vi "SubPanelRef.vi"(0 "reference":refnum<vi>, 11 "error in":errorcluster) -> (4 "reference out":refnum<vi>, 8 "InsertedVI":refnum<vi>, 15 "error out":errorcluster)   [LabVIEW 2016]
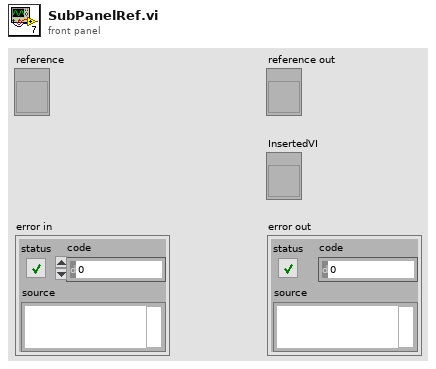
[diagram p1: front panel]
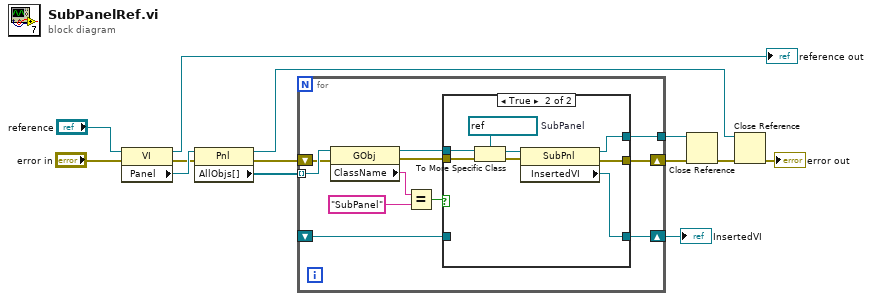
[diagram p0: block diagram]
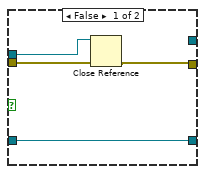
[diagram p2: hidden frame]
diagram:
  n1 = property class="VI"(reference="reference", error in="error in") -> (reference out=→"reference out":refnum<vi>, error out=w9:errorcluster, "Panel"=w13:refnum<vi>)
  n2 = property class="Pnl"(reference=w13, error in=w9) -> (reference out=w4:refnum<vi>, error out=w8:errorcluster, "AllObjs[]"=w12:refnum<vi>[])
  n3 = for {
    tunnel: w12 -> [w24] mode=indexing
    shift-right: [w19] -> w11
    shift-left: _ -> [w18]
    shift-right: [w15] -> w7
    shift-left: w8 -> [w17]
    tunnel: [w14] -> w6
    n4 = property class="GObj"(reference=w24, error in=w17) -> (reference out=w20:refnum<vi>, error out=w16:errorcluster, "ClassName"=w23:string)
    n5 = Equal?(x=w23, y="SubPanel") -> (x = y?=w21:bool)
    n6 = case shown="True" w21 {
      tunnel: w20 -> [w27 w35]
      tunnel: [w28 w33] -> w19
      tunnel: w18 -> [w28 _]
      tunnel: w16 -> [w26 w32]
      tunnel: [w25 w30] -> w15
      tunnel: [_ w29] -> w14
      frame False {
        n7 = Close Reference(reference=w27, error in (no error)=w26) -> (error out=w25:errorcluster)
      }
      frame True {
        w36 = refnum<vi> refnum  # SubPanel
        n8 = To More Specific Class(target class=w36, reference=w35, error in=w32) -> (specific class reference=w34:refnum<vi>, error out=w31:errorcluster)
        n9 = property class="SubPnl"(reference=w34, error in=w31) -> (reference out=w29:refnum<vi>, error out=w30:errorcluster, "InsertedVI"=w33:refnum<vi>)
      }
    }
  }
  "InsertedVI" <- w11
  n10 = Close Reference(reference=w6, error in (no error)=w7) -> (error out=w5:errorcluster)
  n11 = Close Reference(reference=w4, error in (no error)=w5) -> (error out=→"error out":errorcluster)
